vi "PADMINI_BOOL_COLOR_CHANGE.vi"(8 "error in (no error)":errorcluster, 10 "Input Result":string, 11 "Boolean in":refnum<vi>) -> (0 "error out":errorcluster)   [LabVIEW 2017]
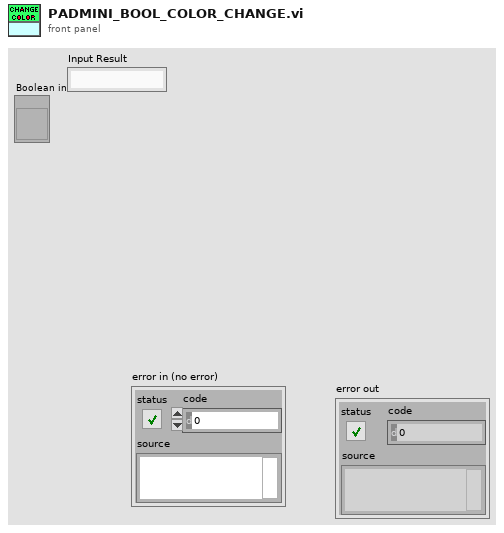
[diagram p1: front panel]
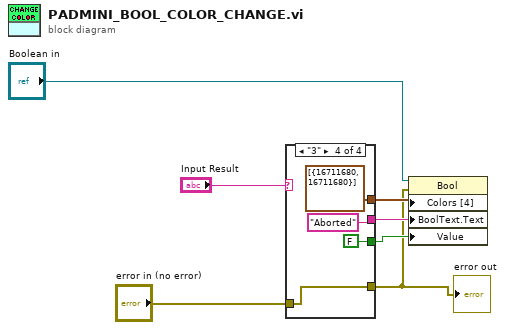
[diagram p0: block diagram]
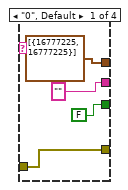
[diagram p2: hidden frame]
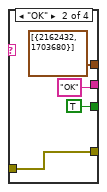
[diagram p3: hidden frame]
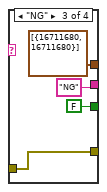
[diagram p4: hidden frame]
diagram:
  n1 = case shown="\"3\"" "Input Result" {
    tunnel: [cluster{u32, u32}[] [{16777225, 16777225}] ("Colors [4]") cluster{u32, u32}[] [{2162432, 1703680}] ("Colors [4]") cluster{u32, u32}[] [{16711680, 16711680}] ("Colors [4]") cluster{u32, u32}[] [{16711680, 16711680}] ("Colors [4]")] -> w5
    tunnel: ["" "OK" "NG" "Aborted"] -> w6
    tunnel: [FALSE TRUE FALSE FALSE] -> w3
    tunnel: [w8 w12 w16 w20] -> w1
    tunnel: "error in (no error)" -> [w8 w12 w16 w20]
    frame "0", Default {
    }
    frame "OK" {
    }
    frame "NG" {
    }
    frame "3" {
    }
  }
  "error out" <- w1
  n2 = property on="Property Node" class="Bool"(reference="Boolean in", error in=w1, "Colors [4]"=w5, "BoolText.Text"=w6, "Value"=w3) -> ()  [unwired: 2 out]
